vi "buff_fgv.vi"(7 "cmd":enum16{"ini", "add"}(ring), 11 "data":dbl) -> (3 "buff":dbl[](array[numeric]))   [LabVIEW 2018]
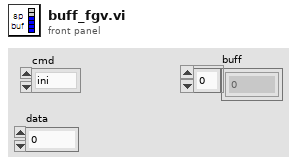
[diagram p1: front panel]
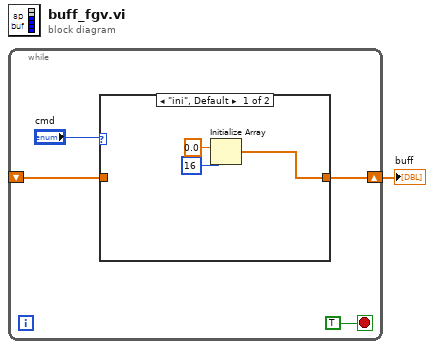
[diagram p0: block diagram]
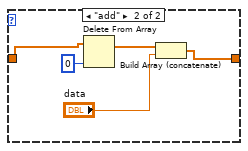
[diagram p2: hidden frame]
diagram:
  n1 = while {
    shift-right: [w3] -> w1
    shift-left: _ -> [w2]
    stop <- TRUE stop-if-true
    n2 = case shown="\"ini\", Default" "cmd" {
      tunnel: [w6 w10] -> w3
      tunnel: w2 -> [_ w11]
      frame "ini", Default {
        n3 = Initialize Array(0.0 ("element"), 16 ("dimension size")) -> (w6:dbl[])
      }
      frame "add" {
        n4 = Delete From Array(array=w11, index=0) -> (array with subset deleted=w13:dbl[])  [unwired: 1 in, 1 out]
        n5 = Build Array (concatenate)(w13, "data") -> (w10:dbl[])
      }
    }
  }
  "buff" <- w1
